vi "Generic command handler.vi"(8 "error in (no error)":errorcluster, 10 "Message in":refnum<class "GenericMessage.lvclass">, 11 "Autofocus in":refnum<class "Autofocus.lvclass">) -> (0 "error out":errorcluster, 2 "value":string, 3 "Autofocus out":refnum<class "Autofocus.lvclass">)   [LabVIEW 2012, in "Autofocus.lvclass"]
doc: "The generic_command_handler processes the command 'generic'. Commands which are not part of the predefined list of commands fall under the 'generic' command for special activity."
uses:
  Autofocus.lvclass
  <vilib>/Distrio/Murmex/GenericMessage/GenericMessage.lvclass
  <vilib>/Distrio/Murmex/Murmex/Murmex.lvclass
  Autofocus.lvclass/Autofocus.ctl
panel:
  # "This method is called when the GENERIC\ntrigger is sent. \n\nOverride this method when your component needs to\nrespond to this trigger. \n\nCall parent for proper implementation"
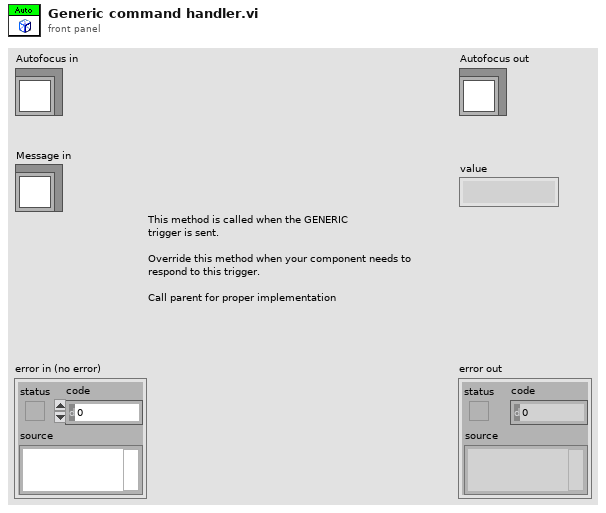
[diagram p1: front panel]
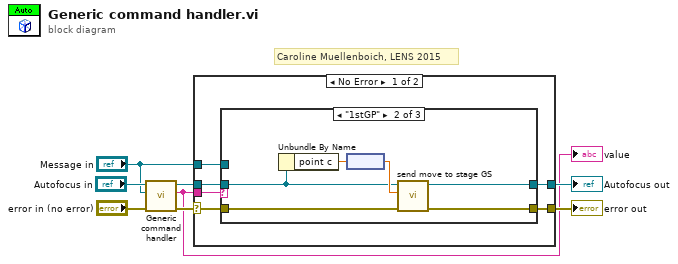
[diagram p0: block diagram]
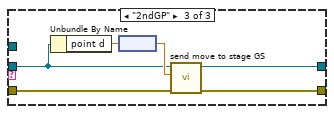
[diagram p3: hidden frame]
diagram:
  # "Caroline Muellenboich, LENS 2015"
  n1 = call-parent "Generic command handler.vi"("error in (no error)"="error in (no error)", "Message in"="Message in", "Murmex in"="Autofocus in") -> ("error out"=w6:errorcluster, "value"=w1:string, "Murmex out"=w5:refnum<class "Autofocus.lvclass">)  [unwired: 6 in]
  "value" <- w1
  n2 = case shown="No Error" w6 {
    selector: w6 -> [w13 w29]
    tunnel: w1 -> [w14 _]
    tunnel: w5 -> [w12 w30]
    tunnel: "Message in" -> [w11 _]
    tunnel: [w10 w29] -> w3
    tunnel: [w9 w30] -> w2
    frame No Error {
      n3 = case shown="\"1stGP\"" w14 {
        tunnel: w13 -> [w16 w22 w28]
        tunnel: w12 -> [w15 w19 w25]
        tunnel: w11 -> [_ _ _]
        tunnel: [w16 w17 w23] -> w10
        tunnel: [w15 w18 w24] -> w9
        frame "False", Default {
        }
        frame "1stGP" {
          n4 = Unbundle By Name(w19) -> ("point c"=w21:dbl)
          n5 = node(w21) -> (w20:dbl[unit])
          n6 = call-dynamic "send move to stage GS.vi"("error in (no error)"=w22, "absolute position"=w20, "Autofocus in"=w19) -> ("error out"=w17:errorcluster, "Autofocus out"=w18:refnum<class "Autofocus.lvclass">)  [unwired: 7 in]
        }
        frame "2ndGP" {
          n7 = Unbundle By Name(w25) -> ("point d"=w27:dbl)
          n8 = node(w27) -> (w26:dbl[unit])
          n9 = call-dynamic "send move to stage GS.vi"("error in (no error)"=w28, "absolute position"=w26, "Autofocus in"=w25) -> ("error out"=w23:errorcluster, "Autofocus out"=w24:refnum<class "Autofocus.lvclass">)  [unwired: 7 in]
        }
      }
    }
    frame Error {
    }
  }
  "error out" <- w3
  "Autofocus out" <- w2
